vi "update.vi"(8 "error in (no error)":errorcluster, 11 "StimulatorDL090727Writer in":refnum<class "StimulatorDL090727Writer.lvclass">) -> (0 "error out":errorcluster, 3 "StimulatorDL090727Writer out":refnum<class "StimulatorDL090727Writer.lvclass">)   [LabVIEW 2010, in "StimulatorDL090727Writer.lvclass"]
uses:
  StimulatorDL090727Writer.lvclass
  common/enumerations/functional_global_action_enum.ctl
  StimulatorDL090727Writer.lvclass/StimulatorDL090727Writer.ctl
  Clock/GenericClock/GenericClock/GenericClock.lvclass
  SignalWriter/GenericSignalWriter/GenericSignalWriter/GenericSignalWriter.lvclass
  StimulatorDL090724Scaffold/StimulatorDL090724Scaffold/Stimulator090724Scaffold.lvclass
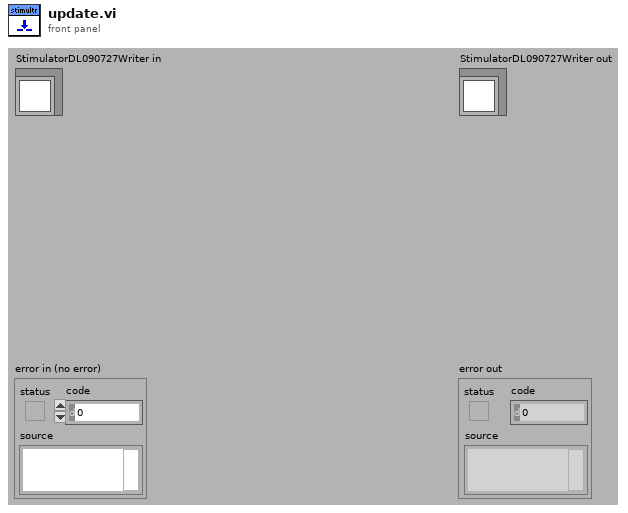
[diagram p1: front panel]
types:
  T1 = typedef "functional_global_action_enum.ctl" = enum16{"get", "set", "reset"}
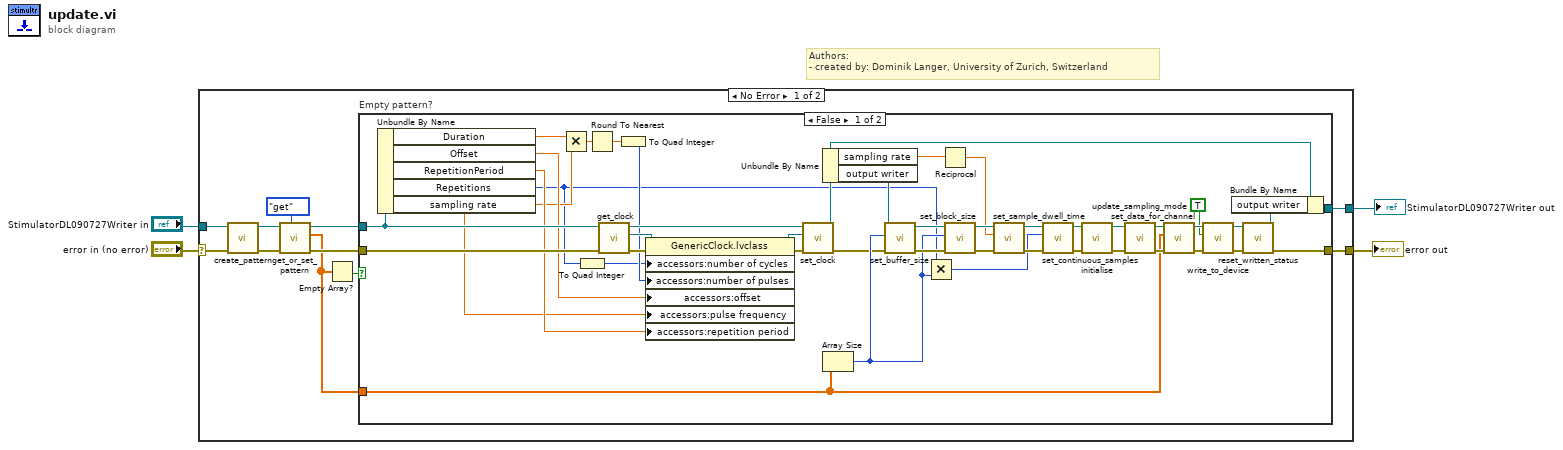
[diagram p0: block diagram]
diagram:
  # "Authors: \n- created by: Dominik Langer, University of Zurich, Switzerland"
  n1 = case shown="No Error" "error in (no error)" {
    selector: "error in (no error)" -> [w6 w62]
    tunnel: "StimulatorDL090727Writer in" -> [w8 w63]
    tunnel: [w14 w62] -> w4
    tunnel: [w13 w63] -> w3
    frame No Error {
      n2 = call-dynamic "create_pattern.vi"("error in (no error)"=w6, "StimulatorDL090727DAQmx in"=w8) -> ("error out"=w5:errorcluster, "StimulatorDL090727DAQmx out"=w7:refnum<class "StimulatorDL090727Writer.lvclass">)  [unwired: 8 out]
      n3 = call-dynamic "get_or_set_pattern.vi"("action"=functional_global_action_enum."get", "error in (no error)"=w5, "Stimulator090724 in"=w7) -> ("error out"=w12:errorcluster, "samples out"=w10:dbl[], "Stimulator090724 out"=w11:refnum<class "StimulatorDL090727Writer.lvclass">)  [unwired: 1 in, 5 out]
      n4 = Empty Array?(array=w10) -> (empty?=w9:bool)
      n5 = case "Empty pattern?" shown="False" w9 {
        tunnel: w10 -> [w45 _]
        tunnel: [w35 w61] -> w14
        tunnel: [w34 w60] -> w13
        tunnel: w12 -> [w28 w61]
        tunnel: w11 -> [w25 w60]
        frame False {
          n6 = Unbundle By Name(w25) -> ("Duration"=w22:dbl[unit], "Offset"=w24:dbl[unit], "RepetitionPeriod"=w23:dbl[unit], "Repetitions"=w16:i32, "sampling rate"=w21:dbl[unit])
          n7 = Multiply(x=w22, y=w21) -> (x*y=w20:dbl)
          n8 = To Quad Integer(1:w16) -> (0:w17:i64)
          n9 = Round To Nearest(number=w20) -> (nearest integer value=w19:dbl)
          n10 = call "get_clock.vi"("error in (no error)"=w28, "Stimulator090724Scaffold in"=w25) -> ("error out"=w30:errorcluster, "clock"=w29:refnum<class "GenericClock.lvclass">, "Stimulator090724Scaffold out"=w33:refnum<class "StimulatorDL090727Writer.lvclass">)  [unwired: 7 in]
          n11 = To Quad Integer(1:w19) -> (0:w18:i64)
          n12 = property class="GenericClock.lvclass"(reference=w29, error in=w30, "accessors:number of cycles"=w17, "accessors:number of pulses"=w18, "accessors:offset"=w24, "accessors:pulse frequency"=w21, "accessors:repetition period"=w23) -> (reference out=w32:refnum<class "GenericClock.lvclass">, error out=w31:errorcluster)
          n13 = call-dynamic "set_clock.vi"("error in (no error)"=w31, "clock"=w32, "Stimulator090724Scaffold in"=w33) -> ("error out"=w27:errorcluster, "Stimulator090724Scaffold out"=w26:refnum<class "StimulatorDL090727Writer.lvclass">)  [unwired: 7 in]
          n14 = Unbundle By Name(w26) -> ("sampling rate"=w41:dbl[unit], "output writer"=w39:refnum<class "GenericSignalWriter.lvclass">)
          n15 = Array Size(array=w45) -> (size(s)=w43:i32)
          n16 = call-dynamic "set_buffer_size.vi"("error in (no error)"=w27, "buffer size (samples)"=w43, "GenericWriteSignals.lvclass in"=w39) -> ("error out"=w59:errorcluster, "GenericWriteSignals.lvclass out"=w58:refnum<class "GenericSignalWriter.lvclass">)  [unwired: 7 out]
          n17 = Multiply(x=w16, y=w43) -> (x*y=w42:i32)
          n18 = Reciprocal(x=w41) -> (1/x=w40:dbl[unit])
          n19 = call "set_block_size.vi"("error in (no error)"=w59, "block size (samples)"=w43, "GenericWriteSignals.lvclass in"=w58) -> ("error out"=w57:errorcluster, "GenericWriteSignals.lvclass out"=w56:refnum<class "GenericSignalWriter.lvclass">)  [unwired: 7 in]
          n20 = call-dynamic "set_sample_dwell_time.vi"("error in (no error)"=w57, "sample dwell time"=w40, "GenericWriteSignals.lvclass in"=w56) -> ("error out"=w53:errorcluster, "GenericWriteSignals.lvclass out"=w50:refnum<class "GenericSignalWriter.lvclass">)  [unwired: 7 in]
          n21 = call-dynamic "set_continuous_samples.vi"("error in (no error)"=w53, "continuous samples"=w42, "GenericWriteSignals.lvclass in"=w50) -> ("error out"=w52:errorcluster, "GenericWriteSignals.lvclass out"=w51:refnum<class "GenericSignalWriter.lvclass">)  [unwired: 7 out]
          n22 = call-dynamic "initialise.vi"("error in (no error)"=w52, "GenericPlugin in"=w51) -> ("error out"=w55:errorcluster, "GenericPlugin out"=w54:refnum<class "GenericSignalWriter.lvclass">)  [unwired: 8 out]
          n23 = call-dynamic "update_sampling_mode.vi"("error in (no error)"=w55, "GenericWriteSignals in"=w54) -> ("error out"=w49:errorcluster, "GenericWriteSignals out"=w46:refnum<class "GenericSignalWriter.lvclass">)  [unwired: 8 out]
          n24 = call-dynamic "set_data_for_channel.vi"("error in (no error)"=w49, "data"=w45, "GenericWriteSignals in"=w46) -> ("error out"=w48:errorcluster, "GenericWriteSignals out"=w47:refnum<class "GenericSignalWriter.lvclass">)  [unwired: 7 out]
          n25 = call-dynamic "write_to_device.vi"("error in (no error)"=w48, "force writing?"=TRUE, "GenericWriteSignals in"=w47) -> ("error out"=w38:errorcluster, "GenericWriteSignals out"=w37:refnum<class "GenericSignalWriter.lvclass">)  [unwired: 7 out]
          n26 = call-dynamic "reset_written_status.vi"("error in (no error)"=w38, "GenericWriteSignals in"=w37) -> ("error out"=w35:errorcluster, "GenericWriteSignals out"=w36:refnum<class "GenericSignalWriter.lvclass">)  [unwired: 8 out]
          n27 = Bundle By Name(cluster=w26, "output writer"=w36) -> (w34:refnum<class "StimulatorDL090727Writer.lvclass">)
        }
        frame True {
        }
      }
    }
    frame Error {
    }
  }
  "error out" <- w4
  "StimulatorDL090727Writer out" <- w3
